vi "RW Controller Settings.vi"(0 "Filepath":path, 2 "Read (F)":bool, 5 "Controller Name":string, 7 "ControlArray In":T1(array[cluster])=[{"Name"="Volt_Direct", "PI Far->Close"=[], "FFinfo"={"FF_m"=0.0, "FF_b"=0.0}, "Limits"={"StepSize"=1e-05, "Max"=10.0, "Min"=0.0, "IndMin"=0.0}}, {"Name"="Volt_Flow", "PI Far->Close"=[], "FFinfo"={"FF_m"=0.0, "FF_b"=0.0}, "Limits"={"StepSize"=1e-05, "Max"=10.0, "Min"=0.0, "IndMin"=0.0}}, {"Name"="Volt_Speed", "PI Far->Close"=[], "FFinfo"={"FF_m"=0.0, "FF_b"=0.0}, "Limits"={"StepSize"=1e-05, "Max"=10.0, "Min"=0.0, "IndMin"=0.0}}, {"Name"="Pres_Direct", "PI Far->Close"=[], "FFinfo"={"FF_m"=0.0, "FF_b"=0.0}, "Limits"={"StepSize"=1e-05, "Max"=10.0, "Min"=0.0, "IndMin"=0.0}}, {"Name"="Pres_Flow", "PI Far->Close"=[], "FFinfo"={"FF_m"=0.0, "FF_b"=0.0}, "Limits"={"StepSize"=1e-05, "Max"=10.0, "Min"=0.0, "IndMin"=0.0}}, {"Name"="Pres_Speed", "PI Far->Close"=[], "FFinfo"={"FF_m"=0.0, "FF_b"=0.0}, "Limits"={"StepSize"=1e-05, "Max"=10.0, "Min"=0.0, "IndMin"=0.0}}, {"Name"="CMD_Direct", "PI Far->Close"=[], "FFinfo"={"FF_m"=0.0, "FF_b"=0.0}, "Limits"={"StepSize"=1e-05, "Max"=10.0, "Min"=0.0, "IndMin"=0.0}}, {"Name"="CMD_Flow", "PI Far->Close"=[], "FFinfo"={"FF_m"=0.0, "FF_b"=0.0}, "Limits"={"StepSize"=1e-05, "Max"=10.0, "Min"=0.0, "IndMin"=0.0}}, {"Name"="CMD_Speed", "PI Far->Close"=[], "FFinfo"={"FF_m"=0.0, "FF_b"=0.0}, "Limits"={"StepSize"=1e-05, "Max"=10.0, "Min"=0.0, "IndMin"=0.0}}], 11 "Error In":errorcluster) -> (8 "ControlArray Out":T1(array[cluster])=[{"Name"="Volt_Direct", "PI Far->Close"=[], "FFinfo"={"FF_m"=0.0, "FF_b"=0.0}, "Limits"={"StepSize"=1e-05, "Max"=10.0, "Min"=0.0, "IndMin"=0.0}}, {"Name"="Volt_Flow", "PI Far->Close"=[], "FFinfo"={"FF_m"=0.0, "FF_b"=0.0}, "Limits"={"StepSize"=1e-05, "Max"=10.0, "Min"=0.0, "IndMin"=0.0}}, {"Name"="Volt_Speed", "PI Far->Close"=[], "FFinfo"={"FF_m"=0.0, "FF_b"=0.0}, "Limits"={"StepSize"=1e-05, "Max"=10.0, "Min"=0.0, "IndMin"=0.0}}, {"Name"="Pres_Direct", "PI Far->Close"=[], "FFinfo"={"FF_m"=0.0, "FF_b"=0.0}, "Limits"={"StepSize"=1e-05, "Max"=10.0, "Min"=0.0, "IndMin"=0.0}}, {"Name"="Pres_Flow", "PI Far->Close"=[], "FFinfo"={"FF_m"=0.0, "FF_b"=0.0}, "Limits"={"StepSize"=1e-05, "Max"=10.0, "Min"=0.0, "IndMin"=0.0}}, {"Name"="Pres_Speed", "PI Far->Close"=[], "FFinfo"={"FF_m"=0.0, "FF_b"=0.0}, "Limits"={"StepSize"=1e-05, "Max"=10.0, "Min"=0.0, "IndMin"=0.0}}, {"Name"="CMD_Direct", "PI Far->Close"=[], "FFinfo"={"FF_m"=0.0, "FF_b"=0.0}, "Limits"={"StepSize"=1e-05, "Max"=10.0, "Min"=0.0, "IndMin"=0.0}}, {"Name"="CMD_Flow", "PI Far->Close"=[], "FFinfo"={"FF_m"=0.0, "FF_b"=0.0}, "Limits"={"StepSize"=1e-05, "Max"=10.0, "Min"=0.0, "IndMin"=0.0}}, {"Name"="CMD_Speed", "PI Far->Close"=[], "FFinfo"={"FF_m"=0.0, "FF_b"=0.0}, "Limits"={"StepSize"=1e-05, "Max"=10.0, "Min"=0.0, "IndMin"=0.0}}], 15 "Error Out":errorcluster)   [LabVIEW 2013]
uses:
  <vilib>/Utility/config.llb/Write Key (Double).vi
  <vilib>/Utility/config.llb/Write Key (String).vi
  <vilib>/Utility/config.llb/Read Key (Double).vi
  <vilib>/Utility/config.llb/Read Key (String).vi
  <vilib>/Utility/config.llb/NI_LVConfig.lvlib
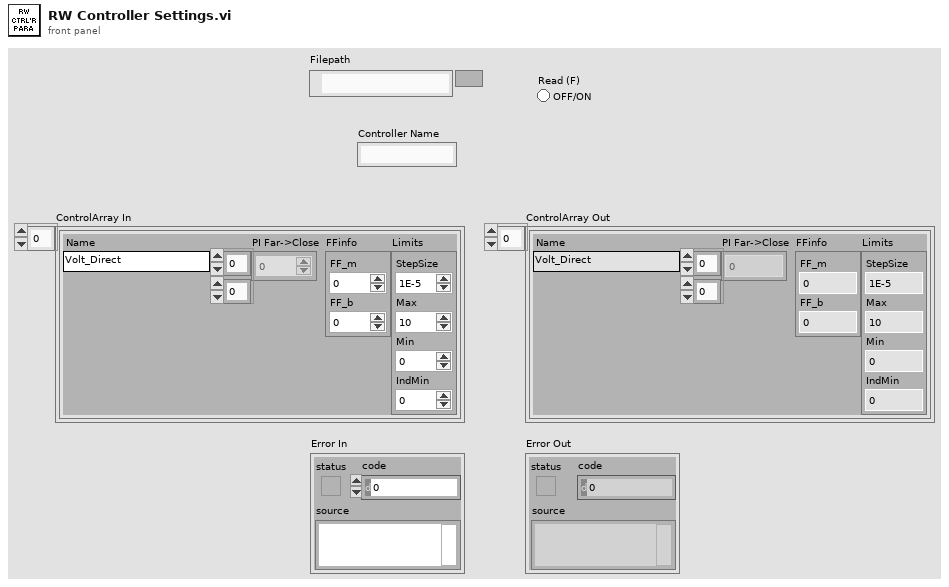
[diagram p1: front panel]
types:
  T1 = cluster{"Name":string, "PI Far->Close":dbl[][], "FFinfo":cluster{"FF_m":dbl, "FF_b":dbl}, "Limits":cluster{"StepSize":dbl, "Max":dbl, "Min":dbl, "IndMin":dbl}}[]
  T2 = typedef "NI_LVConfig.lvlib/Config Data RefNum.ctl" = refnum<k1>
  T3 = cluster{"StepSize":dbl, "Max":dbl, "Min":dbl, "IndMin":dbl}
  T4 = cluster{"value":dbl, "value":dbl, "value":dbl, "value":dbl}
  T5 = cluster{"Name":string, "PI Far->Close":dbl[][], "FFinfo":cluster{"FF_m":dbl, "FF_b":dbl}, "Limits":cluster{"StepSize":dbl, "Max":dbl, "Min":dbl, "IndMin":dbl}}
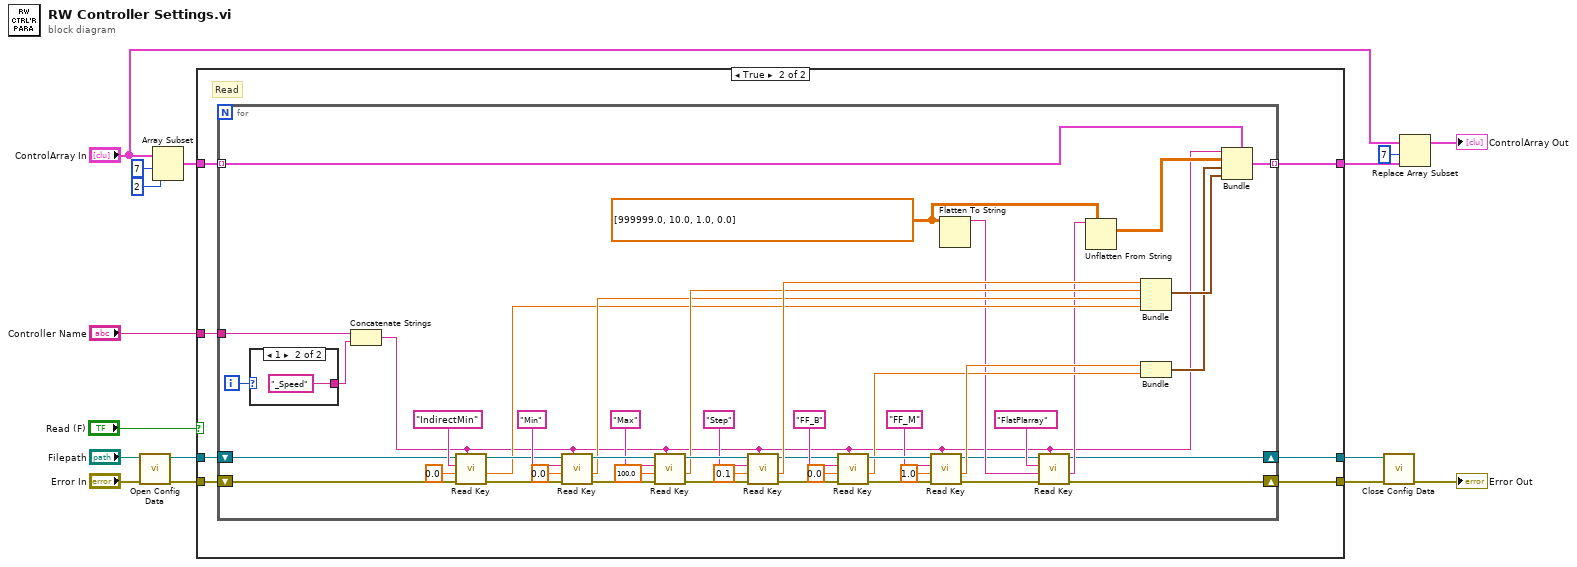
[diagram p0: block diagram]
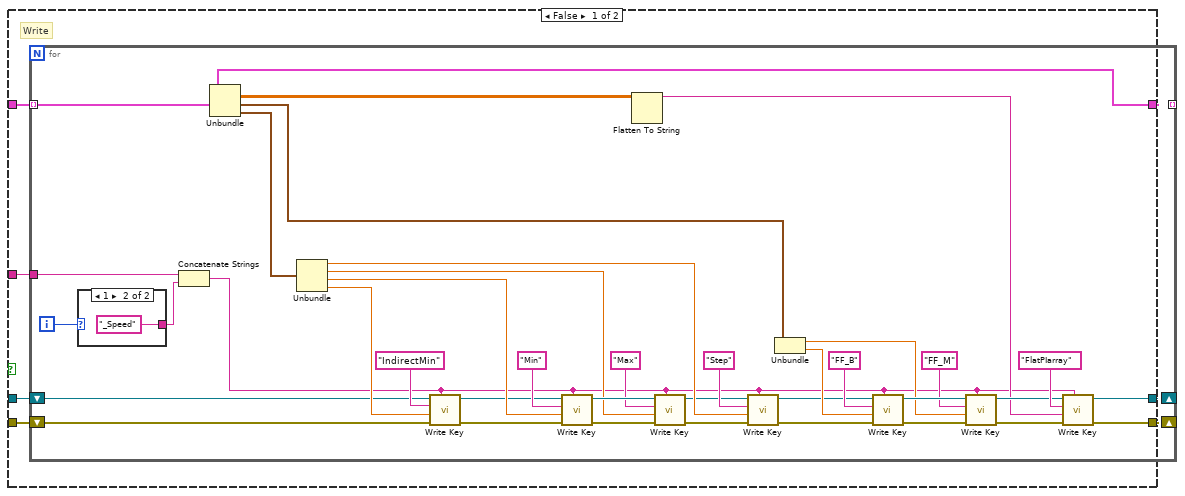
[diagram p2: hidden frame]
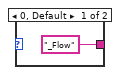
[diagram p3: hidden frame]
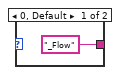
[diagram p4: hidden frame]
diagram:
  n1 = call <vilib>:"Open Config Data.vi"("error in (no error)"="Error In", "configuration file path"="Filepath") -> ("error out"=w10:errorcluster, "refnum"=w11:T2)  [unwired: 7 in, 1 out]
  n2 = Array Subset(array="ControlArray In", index=7, length=2) -> (w12:T1)
  n3 = case shown="True" "Read (F)" {
    tunnel: w11 -> [w23 w69]
    tunnel: w10 -> [w22 w68]
    tunnel: "Controller Name" -> [w17 w64]
    tunnel: w12 -> [w21 w70]
    tunnel: [w20 w67] -> w16
    tunnel: [w19 w66] -> w5
    tunnel: [w18 w65] -> w4
    frame False {
      # "Write"
      n4 = for {
        tunnel: w21 -> [w44] mode=indexing
        shift-right: [w28] -> w19
        shift-left: w23 -> [w34]
        shift-right: [w27] -> w18
        shift-left: w22 -> [w33]
        tunnel: [w44] -> w20 mode=indexing
        tunnel: w17 -> [w42]
        i -> [w41]
        n5 = case shown="1" w41 {
          tunnel: ["_Flow" "_Speed"] -> w43
          frame 0, Default {
          }
          frame 1 {
          }
        }
        n6 = Concatenate Strings(w42, w43) -> (w24:string)
        n7 = Unbundle(w44) -> ("PI Far->Close"=w26:dbl[][], "FFinfo"=w36:cluster{"FF_m":dbl, "FF_b":dbl}, "Limits"=w35:T3)  [unwired: 1 out]
        n8 = Unbundle(w35) -> ("StepSize"=w48:dbl, "Max"=w51:dbl, "Min"=w55:dbl, "IndMin"=w37:dbl)
        n9 = call-poly <vilib>:"Write Key.vi"("section"=w24, "error in (no error)"=w33, "value"=w37, "key"="IndirectMin", "refnum"=w34) -> ("error out"=w39:errorcluster, "refnum out"=w40:T2)  [unwired: 4 in, 1 out]
        n10 = call-poly <vilib>:"Write Key.vi"("section"=w24, "error in (no error)"=w39, "value"=w55, "key"="Min", "refnum"=w40) -> ("error out"=w50:errorcluster, "refnum out"=w53:T2)  [unwired: 4 in, 1 out]
        n11 = Flatten To String(anything=w26) -> (data string=w25:string)  [unwired: 3 in, 2 out]
        n12 = call-poly <vilib>:"Write Key.vi"("section"=w24, "error in (no error)"=w50, "value"=w51, "key"="Max", "refnum"=w53) -> ("error out"=w47:errorcluster, "refnum out"=w46:T2)  [unwired: 4 in, 1 out]
        n13 = call-poly <vilib>:"Write Key.vi"("section"=w24, "error in (no error)"=w47, "value"=w48, "key"="Step", "refnum"=w46) -> ("error out"=w31:errorcluster, "refnum out"=w32:T2)  [unwired: 4 in, 1 out]
        n14 = Unbundle(w36) -> ("FF_m"=w57:dbl, "FF_b"=w60:dbl)
        n15 = call-poly <vilib>:"Write Key.vi"("section"=w24, "error in (no error)"=w31, "value"=w60, "key"="FF_B", "refnum"=w32) -> ("error out"=w58:errorcluster, "refnum out"=w59:T2)  [unwired: 4 in, 1 out]
        n16 = call-poly <vilib>:"Write Key.vi"("section"=w24, "error in (no error)"=w58, "value"=w57, "key"="FF_M", "refnum"=w59) -> ("error out"=w29:errorcluster, "refnum out"=w30:T2)  [unwired: 4 in, 1 out]
        n17 = call-poly <vilib>:"Write Key.vi"("section"=w24, "error in (no error)"=w29, "value"=w25, "key"="FlatPIarray", "refnum"=w30) -> ("error out"=w27:errorcluster, "refnum out"=w28:T2)  [unwired: 4 in, 1 out]
      }
    }
    frame True {
      # "Read"
      n18 = for {
        tunnel: w70 -> [w100] mode=indexing
        shift-right: [w73] -> w66
        shift-left: w69 -> [w75]
        shift-right: [w72] -> w65
        shift-left: w68 -> [w74]
        tunnel: [w99] -> w67 mode=indexing
        tunnel: w64 -> [w97]
        i -> [w98]
        w82 = dbl[][] [[999999.0, 10.0, 1.0, 0.0]]
        n19 = case shown="1" w98 {
          tunnel: ["_Flow" "_Speed"] -> w96
          frame 0, Default {
          }
          frame 1 {
          }
        }
        n20 = Concatenate Strings(w97, w96) -> (w71:string)
        n21 = call-poly <vilib>:"Read Key.vi"("section"=w71, "error in (no error)"=w74, "default value"=0.0, "key"="IndirectMin", "refnum"=w75) -> ("error out"=w88:errorcluster, "value"=w86:dbl, "refnum out"=w89:T2)  [unwired: 3 in, 1 out]
        n22 = call-poly <vilib>:"Read Key.vi"("section"=w71, "error in (no error)"=w88, "default value"=0.0, "key"="Min", "refnum"=w89) -> ("error out"=w115:errorcluster, "value"=w103:dbl, "refnum out"=w113:T2)  [unwired: 3 in, 1 out]
        n23 = call-poly <vilib>:"Read Key.vi"("section"=w71, "error in (no error)"=w115, "default value"=100.0, "key"="Max", "refnum"=w113) -> ("error out"=w114:errorcluster, "value"=w104:dbl, "refnum out"=w112:T2)  [unwired: 3 in, 1 out]
        n24 = call-poly <vilib>:"Read Key.vi"("section"=w71, "error in (no error)"=w114, "default value"=0.1, "key"="Step", "refnum"=w112) -> ("error out"=w76:errorcluster, "value"=w105:dbl, "refnum out"=w77:T2)  [unwired: 3 in, 1 out]
        n25 = call-poly <vilib>:"Read Key.vi"("section"=w71, "error in (no error)"=w76, "default value"=0.0, "key"="FF_B", "refnum"=w77) -> ("error out"=w116:errorcluster, "value"=w101:dbl, "refnum out"=w117:T2)  [unwired: 3 in, 1 out]
        n26 = call-poly <vilib>:"Read Key.vi"("section"=w71, "error in (no error)"=w116, "default value"=1.0, "key"="FF_M", "refnum"=w117) -> ("error out"=w79:errorcluster, "value"=w102:dbl, "refnum out"=w78:T2)  [unwired: 3 in, 1 out]
        n27 = Flatten To String(anything=w82) -> (data string=w83:string)  [unwired: 3 in, 2 out]
        n28 = call-poly <vilib>:"Read Key.vi"("section"=w71, "error in (no error)"=w79, "default value"=w83, "key"="FlatPIarray", "refnum"=w78) -> ("error out"=w72:errorcluster, "value"=w81:string, "refnum out"=w73:T2)  [unwired: 3 in, 1 out]
        n29 = Unflatten From String(type=w82, binary string=w81) -> (value=w80:dbl[][])  [unwired: 3 in, 2 out]
        n30 = Bundle("value"=w105, "value"=w104, "value"=w103, "value"=w86) -> (w85:T4)  [unwired: 1 in]
        n31 = Bundle("value"=w102, "value"=w101) -> (w84:cluster{"value":dbl, "value":dbl})  [unwired: 1 in]
        n32 = Bundle(cluster=w100, "Name"=w71, "PI Far->Close"=w80, "FFinfo"=w84, "Limits"=w85) -> (w99:T5)
      }
    }
  }
  n33 = call <vilib>:"Close Config Data.vi"("error in (no error)"=w4, "refnum"=w5) -> ("error out"=→"Error Out":errorcluster)  [unwired: 8 in, 1 out]
  n34 = Replace Array Subset(array="ControlArray In", new element=w16, index=7) -> (→"ControlArray Out":T1)
